vi "Create TestCase Template Instance_rcf.vi"(8 "error in":errorcluster, 10 "Template Class Path":path, 11 "Application Ref (This Application)":refnum<vi>) -> (0 "error out":errorcluster, 3 "Application Ref":refnum<vi>)   [LabVIEW 2009]
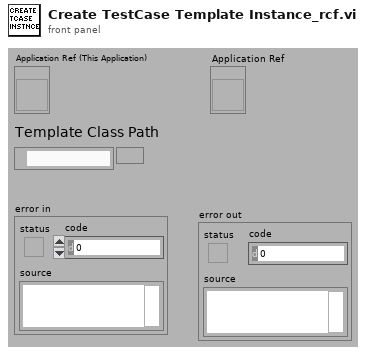
[diagram p1: front panel]
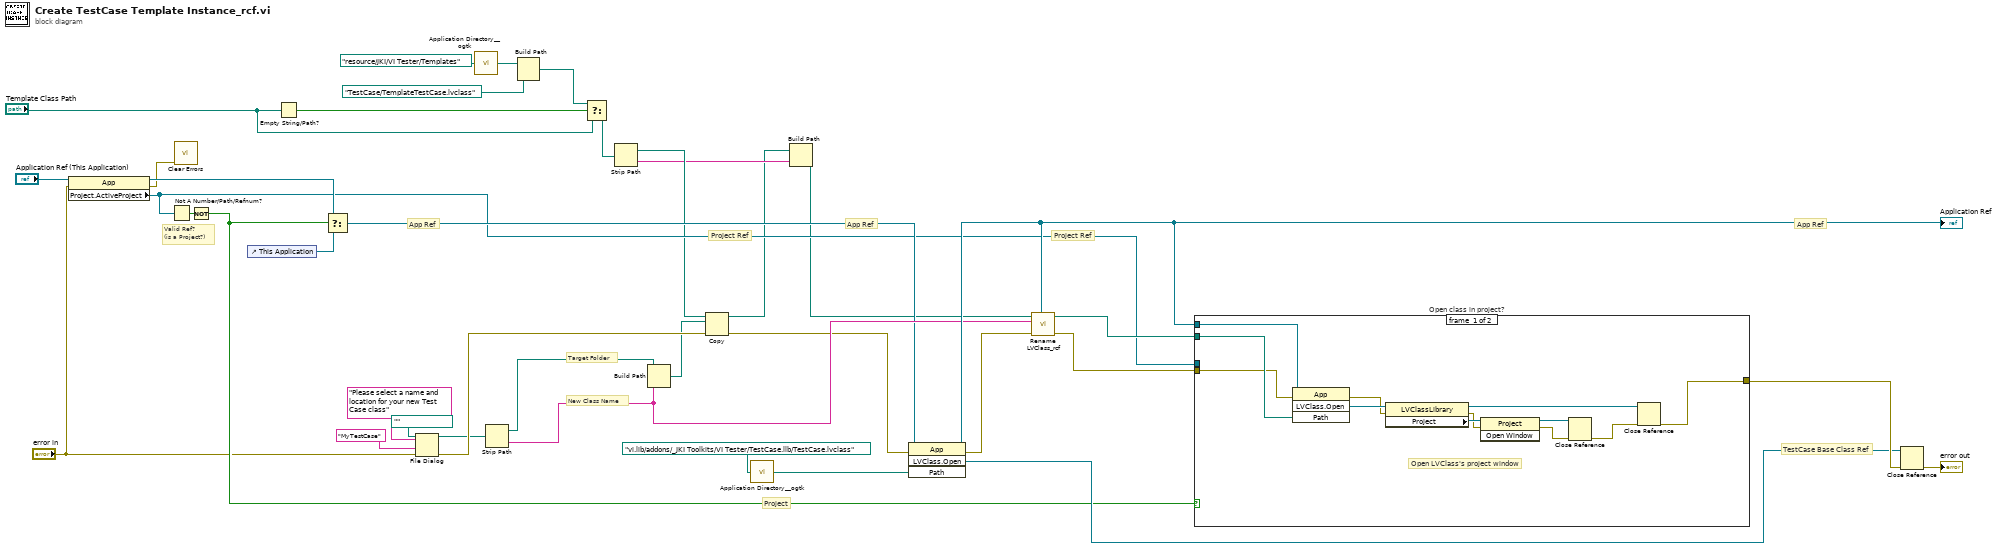
[diagram p0: block diagram]
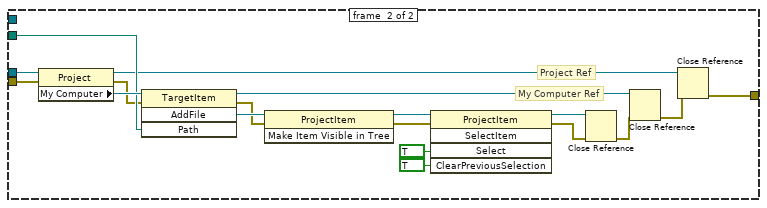
[diagram p2: hidden frame]
diagram:
  # "Project Ref"
  # "App Ref"
  # "Valid Ref?\n(is a Project?)"
  # "TestCase Base Class Ref"
  # "Project"
  # "App Ref"
  # "Project Ref"
  # "App Ref"
  # "Target Folder"
  # "New Class Name"
  n1 = property class="App"(reference="Application Ref (This Application)", error in="error in") -> (reference out=w18:refnum<vi>, error out=w13:errorcluster, "Project.ActiveProject"=w14:refnum<vi>)
  n2 = Not A Number/Path/Refnum?(number/path/refnum=w14) -> (NaN/Path/Refnum?=w20:bool)
  n3 = call <vilib>:"Clear Errors.vi"("error in (no error)"=w13) -> ()  [unwired: 6 in, 1 out]
  n4 = Not(x=w20) -> (.not. x?=w15:bool)
  n5 = control-ref of="This Application"() -> (w19:refnum<vi>)
  n6 = Empty String/Path?(string/path="Template Class Path") -> (empty?=w11:bool)
  n7 = Select(t=w18, s=w15, f=w19) -> (s? t:f=w16:refnum<vi>)
  n8 = File Dialog(7:"Please select a name and location for your new Test Case class" ("prompt"), 8:"error in", 9:"MyTestCase" ("default name"), 11:path "" ("start path")) -> (0:w38:errorcluster, 3:w37:path)  [unwired: 3 in, 2 out]
  n9 = call <userlib>:"Application Directory__ogtk.vi"("Relative path (.)"=path "resource/JKI/VI Tester/Templates") -> ("Application Directory (+ Relative)"=w10:path)
  n10 = Strip Path(path=w37) -> (stripped path=w28:path, name=w29:string)
  n11 = Build Path(base path=w10, name or relative path=path "TestCase/TemplateTestCase.lvclass") -> (appended path=w7:path)
  n12 = Select(t=w7, s=w11, f="Template Class Path") -> (s? t:f=w5:path)
  n13 = Strip Path(path=w5) -> (stripped path=w4:path, name=w3:string)
  n14 = Build Path(base path=w28, name or relative path=w29) -> (appended path=w21:path)
  n15 = Copy(8:w38, 10:w21, 11:w4) -> (0:w24:errorcluster, 3:w2:path)  [unwired: 2 in, 1 out]
  n16 = call <userlib>:"Application Directory__ogtk.vi"("Relative path (.)"=path "vi.lib/addons/_JKI Toolkits/VI Tester/TestCase.llb/TestCase.lvclass") -> ("Application Directory (+ Relative)"=w23:path)
  n17 = Build Path(base path=w2, name or relative path=w3) -> (appended path=w1:path)
  n18 = invoke class="App" method="LVClass.Open"(reference=w16, error in=w24, "Path"=w23) -> (reference out=w35:refnum<vi>, error out=w25:errorcluster, "LVClass.Open"=w32:refnum<vi>)  [unwired: 1 in, 1 out]
  "Application Ref" <- w35
  n19 = call "Rename LVClass_rcf.vi"("App reference"=w35, "error in (no error)"=w25, "New Class Name"=w29, "LVClass Path"=w1) -> ("error out"=w31:errorcluster, "Updated LVClass Path"=w30:path)  [unwired: 6 in]
  n20 = case "Open class in project?" shown="True" w15 {
    tunnel: w30 -> [w48 w67]
    tunnel: w31 -> [w47 w65]
    tunnel: [w45 w60] -> w34
    tunnel: w14 -> [_ w51]
    tunnel: w35 -> [w41 _]
    frame #0 {
      # "Open LVClass's project window"
      n21 = invoke class="App" method="LVClass.Open"(reference=w41, error in=w47, "Path"=w48) -> (error out=w49:errorcluster, "LVClass.Open"=w50:refnum<vi>)  [unwired: 1 in, 2 out]
      n22 = property class="LVClassLibrary"(reference=w50, error in=w49) -> (reference out=w46:refnum<vi>, error out=w43:errorcluster, "Project"=w44:refnum<vi>)
      n23 = invoke class="Project" method="Open Window"(reference=w44, error in=w43) -> (reference out=w42:refnum<vi>, error out=w40:errorcluster)  [unwired: 1 in, 1 out]
      n24 = Close Reference(reference=w42, error in (no error)=w40) -> (error out=w39:errorcluster)
      n25 = Close Reference(reference=w46, error in (no error)=w39) -> (error out=w45:errorcluster)
    }
    frame #1 {
      # "My Computer Ref"
      # "Project Ref"
      n26 = property class="Project"(reference=w51, error in=w65) -> (reference out=w62:refnum<vi>, error out=w66:errorcluster, "My Computer"=w68:refnum<vi>)
      n27 = invoke class="TargetItem" method="AddFile"(reference=w68, error in=w66, "Path"=w67) -> (reference out=w63:refnum<vi>, error out=w58:errorcluster, "AddFile"=w59:refnum<vi>)  [unwired: 1 in, 1 out]
      n28 = invoke class="ProjectItem" method="Make Item Visible in Tree"(reference=w59, error in=w58) -> (reference out=w55:refnum<vi>, error out=w57:errorcluster)  [unwired: 1 in, 1 out]
      n29 = invoke class="ProjectItem" method="SelectItem"(reference=w55, error in=w57, "Select"=TRUE, "ClearPreviousSelection"=TRUE) -> (reference out=w54:refnum<vi>, error out=w56:errorcluster)  [unwired: 1 in, 3 out]
      n30 = Close Reference(reference=w54, error in (no error)=w56) -> (error out=w64:errorcluster)
      n31 = Close Reference(reference=w63, error in (no error)=w64) -> (error out=w61:errorcluster)
      n32 = Close Reference(reference=w62, error in (no error)=w61) -> (error out=w60:errorcluster)
    }
  }
  n33 = Close Reference(reference=w32, error in (no error)=w34) -> (error out=→"error out":errorcluster)
